vi "Sub VI-X (t).vi"(8 "error in":errorcluster, 10 "t":dbl, 11 "K":dbl) -> (0 "error out":errorcluster, 3 "x (t)":dbl)   [LabVIEW 2024]
doc: "Use this SubVI to create a wave of\nx(t)=exp(-(t-k)^2) this formula."
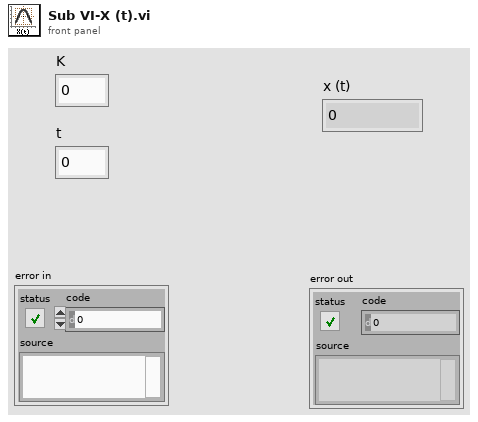
[diagram p1: front panel]
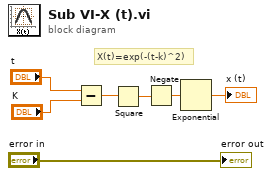
[diagram p0: block diagram]
diagram:
  # "X(t)=exp(-(t-k)^2)"
  n1 = Subtract(x="t", y="K") -> (x-y=w3:dbl)
  n2 = Square(x=w3) -> (x^2=w2:dbl)
  n3 = Negate(x=w2) -> (-x=w1:dbl)
  n4 = Exponential(1:w1) -> (0:→"x (t)":dbl)
  "error out" <- "error in"
